vi "Do.vi"(8 "error in (no error)":errorcluster, 10 "Actor in":refnum<class "Actor.lvclass">, 11 "New image Msg":refnum<class "New image Msg.lvclass">) -> (0 "error out":errorcluster, 2 "Actor out":refnum<class "Actor.lvclass">)   [LabVIEW 2014, in "Camera Tester.lvlib" / "New image Msg.lvclass"]
doc: "(<B>Filename</B>: Actor Framework.lvlib:Message.lvclass:Do.vi)\n\nDefines what a message does when it is received by an actor. Generally, a message instructs an actor to invoke one of its methods. By default, this method does nothing. A child class must override it to define behavior. Create a child class by using the Actor Framework Message Maker dialog box."
uses:
  New image Msg.lvclass
  <vilib>/ActorFramework/Actor/Actor.lvclass
  Camera Tester/Camera Tester.lvclass
  Camera Actor/Camera Actor Messages/New Image Msg/New Image Msg.lvclass/New Image Msg.ctl
  Camera Actor/Camera Actor Messages/New Image Msg/New Image Msg.lvclass
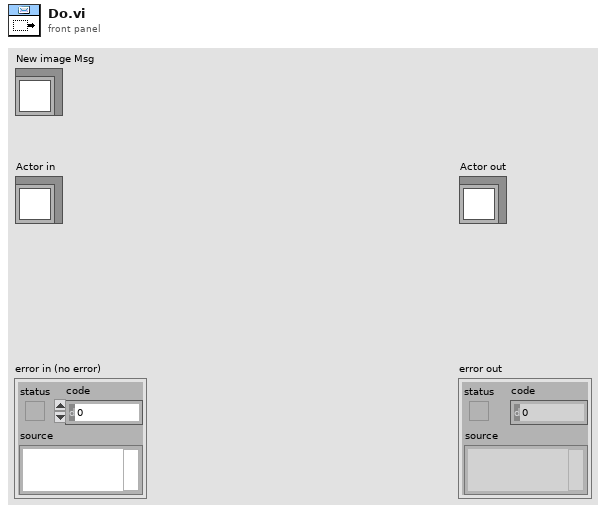
[diagram p1: front panel]
types:
  T1 = typedef "IMAQ Image.ctl" = refnum<image>
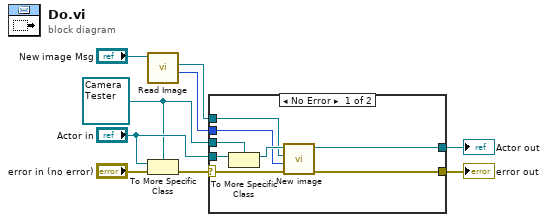
[diagram p0: block diagram]
diagram:
  w2 = refnum<class "Camera Tester.lvclass"> refnum ("Actor in")
  n1 = call "Read Image.vi"("New Image Msg in"="New image Msg") -> ("Buffer Number"=w9:u32, "Image"=w8:T1)  [unwired: 7 in, 2 out]
  n2 = To More Specific Class(target class=w2, reference="Actor in", error in="error in (no error)") -> (error out=w7:errorcluster)  [unwired: 1 out]
  n3 = case shown="No Error" w7 {
    selector: w7 -> [w15 w19]
    tunnel: [w17 w19] -> w3
    tunnel: [w16 w18] -> w4
    tunnel: "Actor in" -> [w14 w18]
    tunnel: w2 -> [w13 _]
    tunnel: w8 -> [w11 _]
    tunnel: w9 -> [w10 _]
    frame No Error {
      n4 = To More Specific Class(target class=w13, reference=w14) -> (specific class reference=w12:refnum<class "Camera Tester.lvclass">)  [unwired: 1 in, 1 out]
      n5 = call-dynamic "New image.vi"("error in (no error)"=w15, "Buffer Number"=w10, "Image"=w11, "Camera Tester in"=w12) -> ("error out"=w17:errorcluster, "Camera Tester out"=w16:refnum<class "Camera Tester.lvclass">)  [unwired: 6 in]
    }
    frame Error {
      # "If type check fails, pass the original object out again."
    }
  }
  "error out" <- w3
  "Actor out" <- w4
